vi "WritebyRef.vi"   [LabVIEW 2019]
doc: "Écrit une valeur dans le contrôle spécifié par refnum. Les valeurs accepté sont soit numérique ou booléenne"
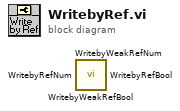
[diagram p0: block diagram]
diagram:
  n1 = call <userlib>:"WritebyWeakRefBool.vi"() -> ()  [unwired: 11 in, 1 out]
  n2 = call <userlib>:"WritebyWeakRefNum.vi"() -> ()  [unwired: 11 in, 1 out]
  n3 = call <userlib>:"WritebyRefNum.vi"() -> ()  [unwired: 11 in, 1 out]
  n4 = call <userlib>:"WritebyRefBool.vi"() -> ()  [unwired: 11 in, 1 out]
